vi "batch-format-converter.vi"() -> ()   [LabVIEW 2017]
uses:
  NHMFL_Core/Libraries/File/File Format Converter/Format Converter Configuration.ctl
panel:
  in  "File":path=path "/Users/arkady/Desktop/Dropbox/local_data/gyro-LANL-Dec2017"
  in  "Configuration":T1={"New start time"=nan, "New end time"=nan, "Output file format"=enum."ASCII", "Save ASCII column names"=TRUE, "Prepend binary array size"=FALSE, "buffer size (-1: all)"=100000, "Channels"=["Time", "Cryo-Con 22C (5) A", "Cryo-Con 22C (5) B", "IPS120 (COM1) Field", "Freq"], "Group"="p", "New dt"=nan} {"buffer size (-1: all)" format="%.0p"; "New start time" format="%#_10p"}
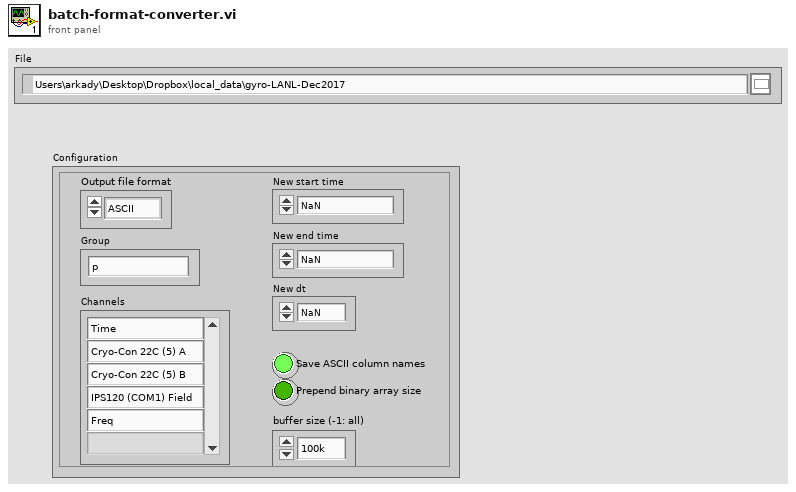
[diagram p1: front panel]
types:
  T1 = typedef "Format Converter Configuration.ctl" = cluster{"New start time":dbl, "New end time":dbl, "Output file format":enum16{"ASCII", "BINARY", "TDMS"}, "Save ASCII column names":bool, "Prepend binary array size":bool, "buffer size (-1: all)":i64, "Channels":string[], "Group":string, "New dt":dbl}
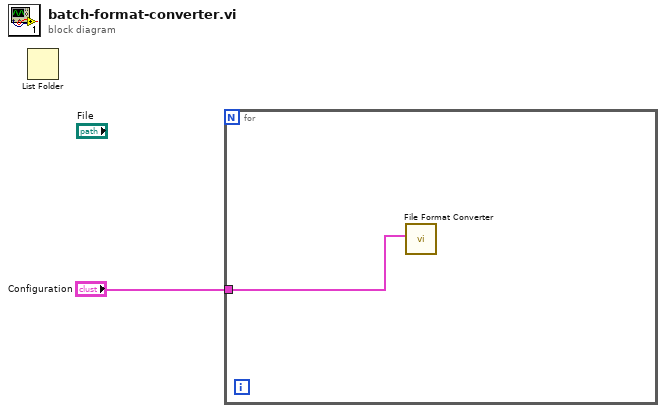
[diagram p0: block diagram]
diagram:
  n1 = List Folder() -> ()  [unwired: 4 in, 4 out]
  n2 = for {
    tunnel: "Configuration" -> [w2]
    n3 = call "File Format Converter.vi"("Configuration"=w2) -> ()  [unwired: 8 in, 3 out]
  }
